vi "posEstByVelPlan.vi"(8 "error in (no error)":errorcluster, 10 "NavigationTeam":refnum<class "Ally.lvclass">, 11 "Ally in":refnum<class "Ally.lvclass">) -> (0 "error out":errorcluster, 3 "Ally out":refnum<class "Ally.lvclass">)   [LabVIEW 2021, in "Ally.lvclass"]
uses:
  Ally.lvclass
  D:/RoboIme/horie/SSL_AI/Team_class/Team.lvclass
  Team_class/Team.lvclass/Team.ctl
  Object_class/Object.lvclass/Object.ctl
  Robot_class/Robot.lvclass/Robot.ctl
  <vilib>/Analysis/coordinate.llb/2D Cartesian Coordinate Rotation (Scalar).vi
  Object_class/Read position(x,y).vi
  Robot_class/Read id.vi
  Robot_class/Read orientation.vi
  Team_class/Read RobotRef.vi
  Team_class/Write RobotRef.vi
  Robot_class/Robot.lvclass
  D:/RoboIme/horie/SSL_AI/Object_class/Object.lvclass
  Utilities_class/Utilities.lvclass
  <vilib>/Analysis/NI_AALPro.lvlib
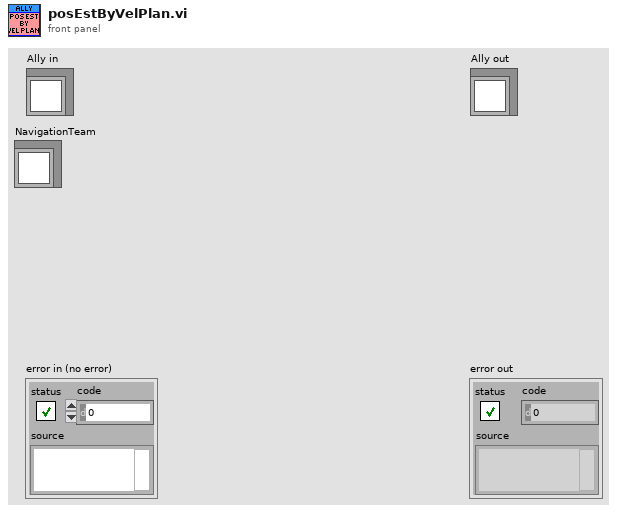
[diagram p1: front panel]
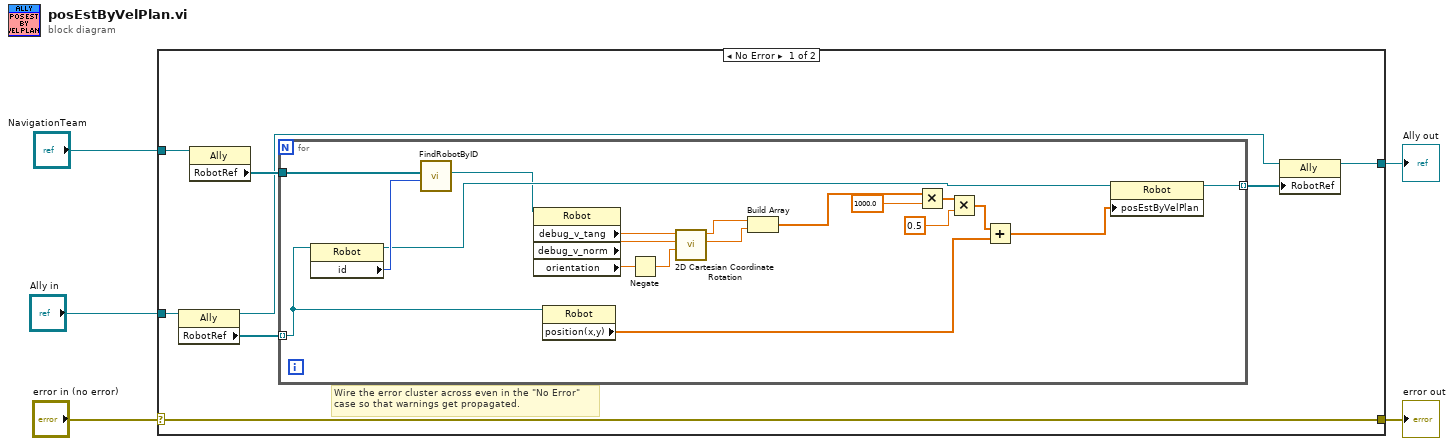
[diagram p0: block diagram]
diagram:
  n1 = case shown="No Error" "error in (no error)" {
    selector: "error in (no error)" -> [w13 w34]
    tunnel: [w13 w34] -> w4
    tunnel: [w6 w33] -> w2
    tunnel: "Ally in" -> [w12 w33]
    tunnel: "NavigationTeam" -> [w10 _]
    frame No Error {
      # "Wire the error cluster across even in the \"No Error\"\ncase so that warnings get propagated."
      n2 = property class="Ally"(reference=w12) -> (reference out=w7:refnum<class "Ally.lvclass">, "RobotRef"=w11:refnum<class "Robot.lvclass">[])  [unwired: 1 in, 1 out]
      n3 = property class="Ally"(reference=w10) -> ("RobotRef"=w9:refnum<class "Robot.lvclass">[])  [unwired: 1 in, 2 out]
      n4 = for {
        tunnel: w11 -> [w17] mode=indexing
        tunnel: w9 -> [w32]
        tunnel: [w29] -> w8 mode=indexing
        n5 = property class="Robot"(reference=w17) -> (reference out=w30:refnum<class "Robot.lvclass">, "id"=w31:i32)  [unwired: 1 in, 1 out]
        n6 = call "FindRobotByID.vi"("id"=w31, "RobotRef"=w32) -> ("Robot"=w28:refnum<class "Robot.lvclass">)  [unwired: 6 in, 3 out]
        n7 = property class="Robot"(reference=w28) -> ("debug_v_tang"=w23:dbl, "debug_v_norm"=w22:dbl, "orientation"=w14:dbl)  [unwired: 1 in, 2 out]
        n8 = property class="Robot"(reference=w17) -> ("position(x,y)"=w16:dbl[])  [unwired: 1 in, 2 out]
        n9 = Negate(x=w14) -> (-x=w15:dbl)
        n10 = call-poly <vilib>:"2D Cartesian Coordinate Rotation.vi"("theta"=w15, "y"=w22, "x"=w23) -> ("y out"=w20:dbl, "x out"=w21:dbl)  [unwired: 6 in, 1 out]
        n11 = Build Array(w21, w20) -> (w19:dbl[])
        n12 = Multiply(x=w19, y=1000.0) -> (x*y=w25:dbl[])
        n13 = Multiply(x=w25, y=0.5) -> (x*y=w26:dbl[])
        n14 = Add(x=w26, y=w16) -> (x+y=w18:dbl[])
        n15 = property class="Robot"(reference=w30, "posEstByVelPlan"=w18) -> (reference out=w29:refnum<class "Robot.lvclass">)  [unwired: 1 in, 1 out]
      }
      n16 = property class="Ally"(reference=w7, "RobotRef"=w8) -> (reference out=w6:refnum<class "Ally.lvclass">)  [unwired: 1 in, 1 out]
    }
    frame Error {
    }
  }
  "error out" <- w4
  "Ally out" <- w2
